vi "Write Index Rect.vi"(5 "Index Rect":T1, 9 "Array in":refnum<class "Array.lvclass">) -> (3 "Array out":refnum<class "Array.lvclass">)   [LabVIEW 2014, in "Raspberry Pi Compatible Compiler for LabVIEW.lvlib" / "Array.lvclass"]
uses:
  Array.lvclass
  <vilib>/Utility/miscctls.llb/LVRectTypeDef.ctl
  Array.lvclass/Array.ctl
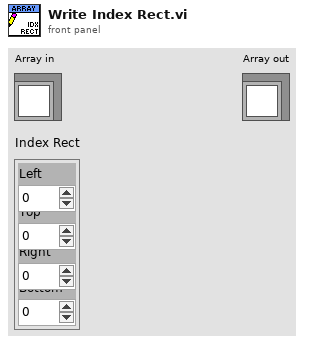
[diagram p1: front panel]
types:
  T1 = typedef "LVRectTypeDef.ctl" = cluster{"Left":i16, "Top":i16, "Right":i16, "Bottom":i16}
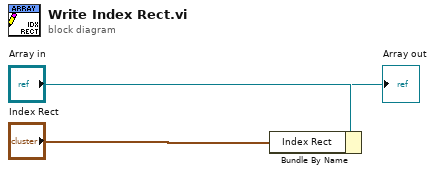
[diagram p0: block diagram]
diagram:
  n1 = Bundle By Name(cluster="Array in", "Index Rect"="Index Rect") -> (→"Array out":refnum<class "Array.lvclass">)
